vi "test PHD Ultra pump.vi"() -> ()   [LabVIEW 2017]
uses:
  <instrlib>/Harvard Apparatus PHD Ultra Series/Harvard Apparatus PHD Ultra Series.lvlib
panel:
  in  "Pump 1 COM":refnum<visa-resource-name>="COM12"
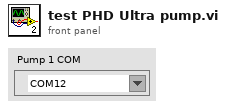
[diagram p1: front panel]
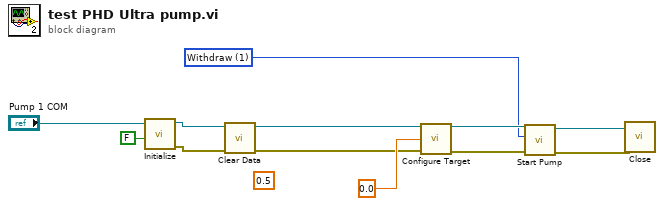
[diagram p0: block diagram]
diagram:
  (unwired) 0.5 ("Flow Rate (5.00)")
  w1 = u16 1 items=["Infuse", "Withdraw"] ("Pump Direction (0:Infuse)")
  n1 = call <instrlib>:"Initialize.vi"("ID Query (True)"=FALSE, "VISA resource name"="Pump 1 COM") -> ("error out"=w11:errorcluster, "VISA resource name out"=w12:refnum<visa-resource-name>)  [unwired: 8 in]
  n2 = call <instrlib>:"Clear Data.vi"("error in (no error)"=w11, "VISA resource name"=w12) -> ("error out"=w2:errorcluster, "VISA resource name out"=w3:refnum<visa-resource-name>)  [unwired: 8 in]
  n3 = call <instrlib>:"Configure Target.vi"("VISA resource name"=w3, "Target Value (5.00)"=0.0, "error in (no error)"=w2) -> ("VISA resource name out"=w10:refnum<visa-resource-name>, "error out"=w9:errorcluster)  [unwired: 11 in]
  n4 = call <instrlib>:"Start Pump.vi"("error in (no error)"=w9, "Run Direction (0:Infuse)"=w1, "VISA resource name"=w10) -> ("error out"=w7:errorcluster, "VISA resource name out"=w8:refnum<visa-resource-name>)  [unwired: 7 in]
  n5 = call <instrlib>:"Close.vi"("error in (no error)"=w7, "VISA resource name"=w8) -> ()  [unwired: 9 in, 1 out]
